vi "Simple Read.vi"(4 "Abs_Boolean_1D.lvclass":refnum<class "Abs_Boolean_1D.lvclass">) -> (1 "Boolean 1D":T1[](array[typedef]))   [LabVIEW 2021, in "Abs_Boolean_1D.lvclass"]
uses:
  Abs_Boolean_1D.lvclass
  Support/Element Type.ctl
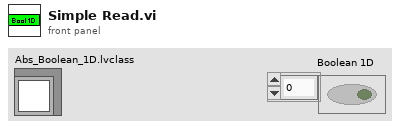
[diagram p1: front panel]
types:
  T1 = typedef "Abs_Boolean_1D.lvclass/Element Type.ctl" = bool
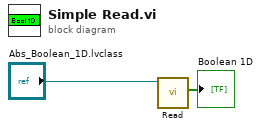
[diagram p0: block diagram]
diagram:
  n1 = call-dynamic "Read.vi"("Boolean in"="Abs_Boolean_1D.lvclass") -> ("Boolean 1D"=→"Boolean 1D":T1[])  [unwired: 8 in, 2 out]
